vi "Teleop[Conflict 1].vi"(10 "Match Info":T1={"Autonomous Elapsed Seconds"=0.0, "TeleOp Elapsed Seconds"=0.0, "Disabled Elapsed Seconds"=0.0, "Visited Autonomous"=FALSE, "Visited TeleOp"=FALSE, "Visited Disabled"=FALSE, "Autonomous Settings"={"Autonomous Style"=enum."Independent", "VI Refnum"=refnum}}, 11 "Call Context":T2) -> ()   [LabVIEW 2016]
doc: "This VI is called for each TeleOp packet received from the DS where the robot is not disabled. It is often used to read from the joysticks and update I/O or to update setpoints for timed control loops. It should complete and return within 20 milliseconds or it may miss DS packets."
uses:
  <vilib>/Rock Robotics/WPI/DriverStation/WPI_DriverStationDerivedRobotMode.ctl
  <vilib>/Rock Robotics/WPI/DriverStation/WPI_DriverStationMatch Info.ctl
  <vilib>/Rock Robotics/Network Tables/NT Read Boolean.vi
  <vilib>/Rock Robotics/Network Tables/NT Read Number.vi
  <vilib>/Rock Robotics/WPI/Utilities/WPI_GetSetVariantRefNum.vi
  <vilib>/Rock Robotics/Network Tables/NT Write Boolean.vi
  <vilib>/Rock Robotics/Network Tables/NT Write Number.vi
  <vilib>/Rock Robotics/Network Tables/NT Write Boolean Array.vi
  <vilib>/Rock Robotics/Network Tables/NT Write Numeric Array.vi
  <vilib>/Rock Robotics/WPI/Solenoid/Deprecated/WPI_SolenoidSetBool.vi
  PDP Currents Variable.vi
panel:
  out "all currents (A) 2":dbl[](array[numeric])
  out "all currents (A)":dbl[](array[numeric])
  out "Enabled":bool
  out "Compressor Running":bool
  out "Sample Slider 0":dbl(slide) scale=0.0..5.0
  out "Sample Boolean 1":bool
  out "Sample Boolean 0":bool
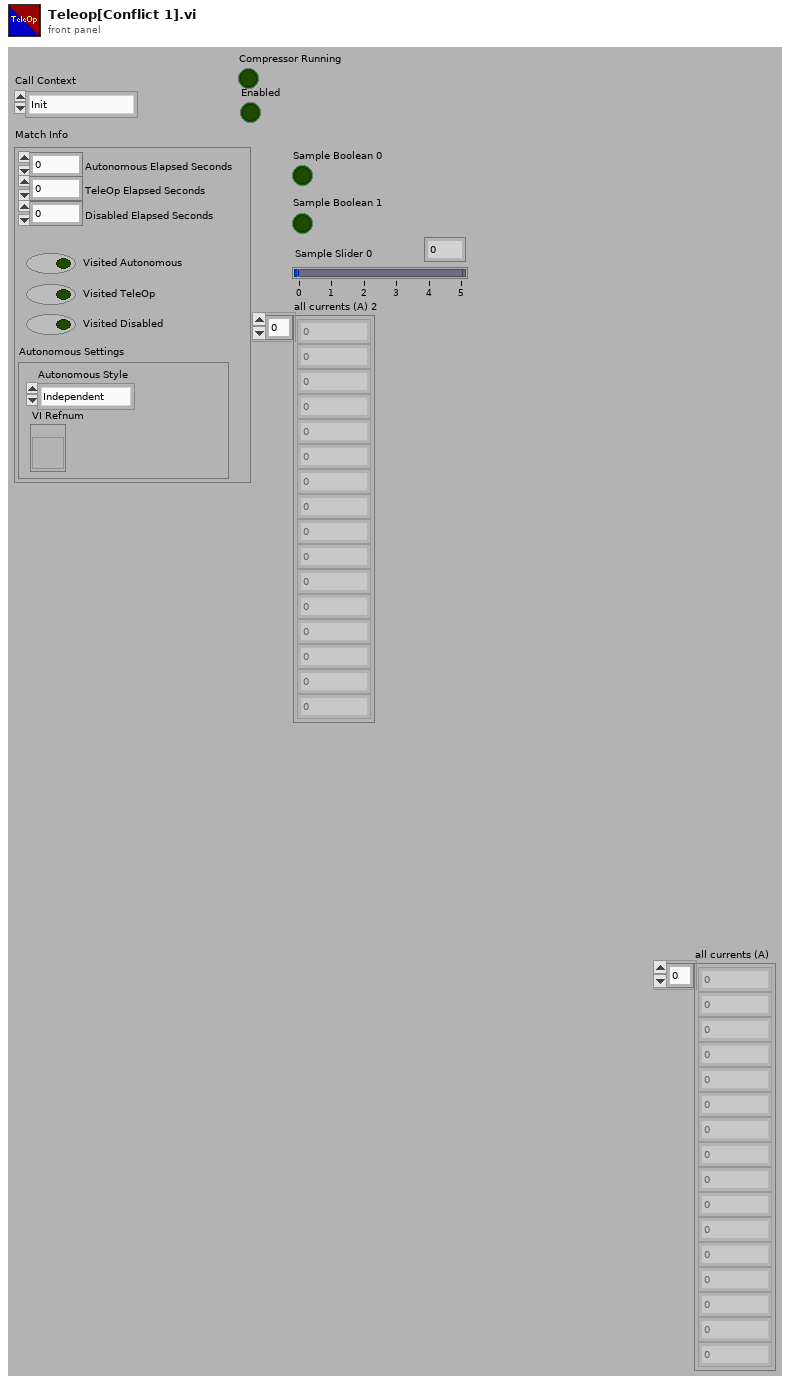
[diagram p1: front panel]
types:
  T1 = typedef "WPI_DriverStationMatch Info.ctl" = cluster{"Autonomous Elapsed Seconds":dbl, "TeleOp Elapsed Seconds":dbl, "Disabled Elapsed Seconds":dbl, "Visited Autonomous":bool, "Visited TeleOp":bool, "Visited Disabled":bool, "Autonomous Settings":cluster{"Autonomous Style":enum16{"Iterative", "Independent"}, "VI Refnum":refnum<vi>}}
  T2 = typedef "WPI_DriverStationDerivedRobotMode.ctl" = enum16{"Init", "Execute", "Stop"}
  T3 = typedef "WPI_JoystickDevRef.ctl" = cluster{"Device":T4}
  T4 = typedef "WPI_JoystickDeviceEnum.ctl" = enum16{"USB 0", "USB 1", "USB 2", "USB 3", "USB 4", "USB 5"}
  T5 = typedef "WPI_CompressorDevRef.ctl" = cluster{"DevStatus":errorcluster, "Pneumatics Control Module":u8}
  T6 = typedef "WPI_SolenoidDevRef.ctl" = cluster{"DevStatus":errorcluster, "Pneumatics Control Module":u8, "Forward Solenoid Channel":T7, "Reverse Solenoid Channel":T7}
  T7 = typedef "WPI_SolenoidChannel.ctl" = enum8{"Solenoid 0", "Solenoid 1", "Solenoid 2", "Solenoid 3", "Solenoid 4", "Solenoid 5", "Solenoid 6", "Solenoid 7", "Invalid"}
  T8 = typedef "WPI_SwitchDevRef.ctl" = cluster{"DevStatus":errorcluster, "DIO Channel":T9, "CntIndex":T10, "Normally Closed":bool}
  T9 = typedef "FPGA_DIOChannel.ctl" = enum8{"DIO 0", "DIO 1", "DIO 2", "DIO 3", "DIO 4", "DIO 5", "DIO 6", "DIO 7", "DIO 8", "DIO 9", "DIO MXP 0", "DIO MXP 1", "DIO MXP 2", "DIO MXP 3", "DIO MXP 4", "DIO MXP 5", "DIO MXP 6", "DIO MXP 7", "DIO MXP 8", "DIO MXP 9", "DIO MXP 10", "DIO MXP 11", "DIO MXP 12", "DIO MXP 13", "DIO MXP 14", "DIO MXP 15", "SPI Port CS1", "SPI Port CS2", "SPI Port CS3", "SPI Port MISO", "SPI Port MOSI", "Invalid"}
  T10 = typedef "FPGA_CounterCtrSystemIndex.ctl" = enum8{"Ctr 0", "Ctr 1", "Ctr 2", "Ctr 3", "Ctr 4", "Ctr 5", "Ctr 6", "Ctr 7", "Invalid"}
  T11 = typedef "WPI_MotorControlDeviceRef.ctl" = cluster{"DeviceStatus":errorcluster, "Type":T12, "PWM":cluster{"PWM Channel":T13, "DeadBand":T14}, "CAN":cluster{"Device Number":u8, "SetOutput VI Ref":variant, "GetOutput VI Ref":variant, "Enable VI Ref":variant, "Disable VI Ref":variant, "Data":variant}, "Invert":bool}
  T12 = typedef "WPI_MotorControlType.ctl" = enum16{"PWM", "CAN"}
  T13 = typedef "FPGA_DIOPWMChannel.ctl" = enum8{"PWM 0", "PWM 1", "PWM 2", "PWM 3", "PWM 4", "PWM 5", "PWM 6", "PWM 7", "PWM 8", "PWM 9", "PWM MXP 0", "PWM MXP 1", "PWM MXP 2", "PWM MXP 3", "PWM MXP 4", "PWM MXP 5", "PWM MXP 6", "PWM MXP 7", "PWM MXP 8", "PWM MXP 9", "Invalid"}
  T14 = typedef "WPI_PWMDeadband.ctl" = cluster{"Name":string, "maxPositivePwm":i32, "minPositivePwm":i32, "centerPwm":i32, "maxNegativePwm":i32, "minNegativePwm":i32, "angularRange":u16}
  T15 = typedef "WPI_RobotDriveDevRef.ctl" = cluster{"DevStatus":errorcluster, "Motors[]":T11[], "Square Inputs":bool, "Max Output":dbl}
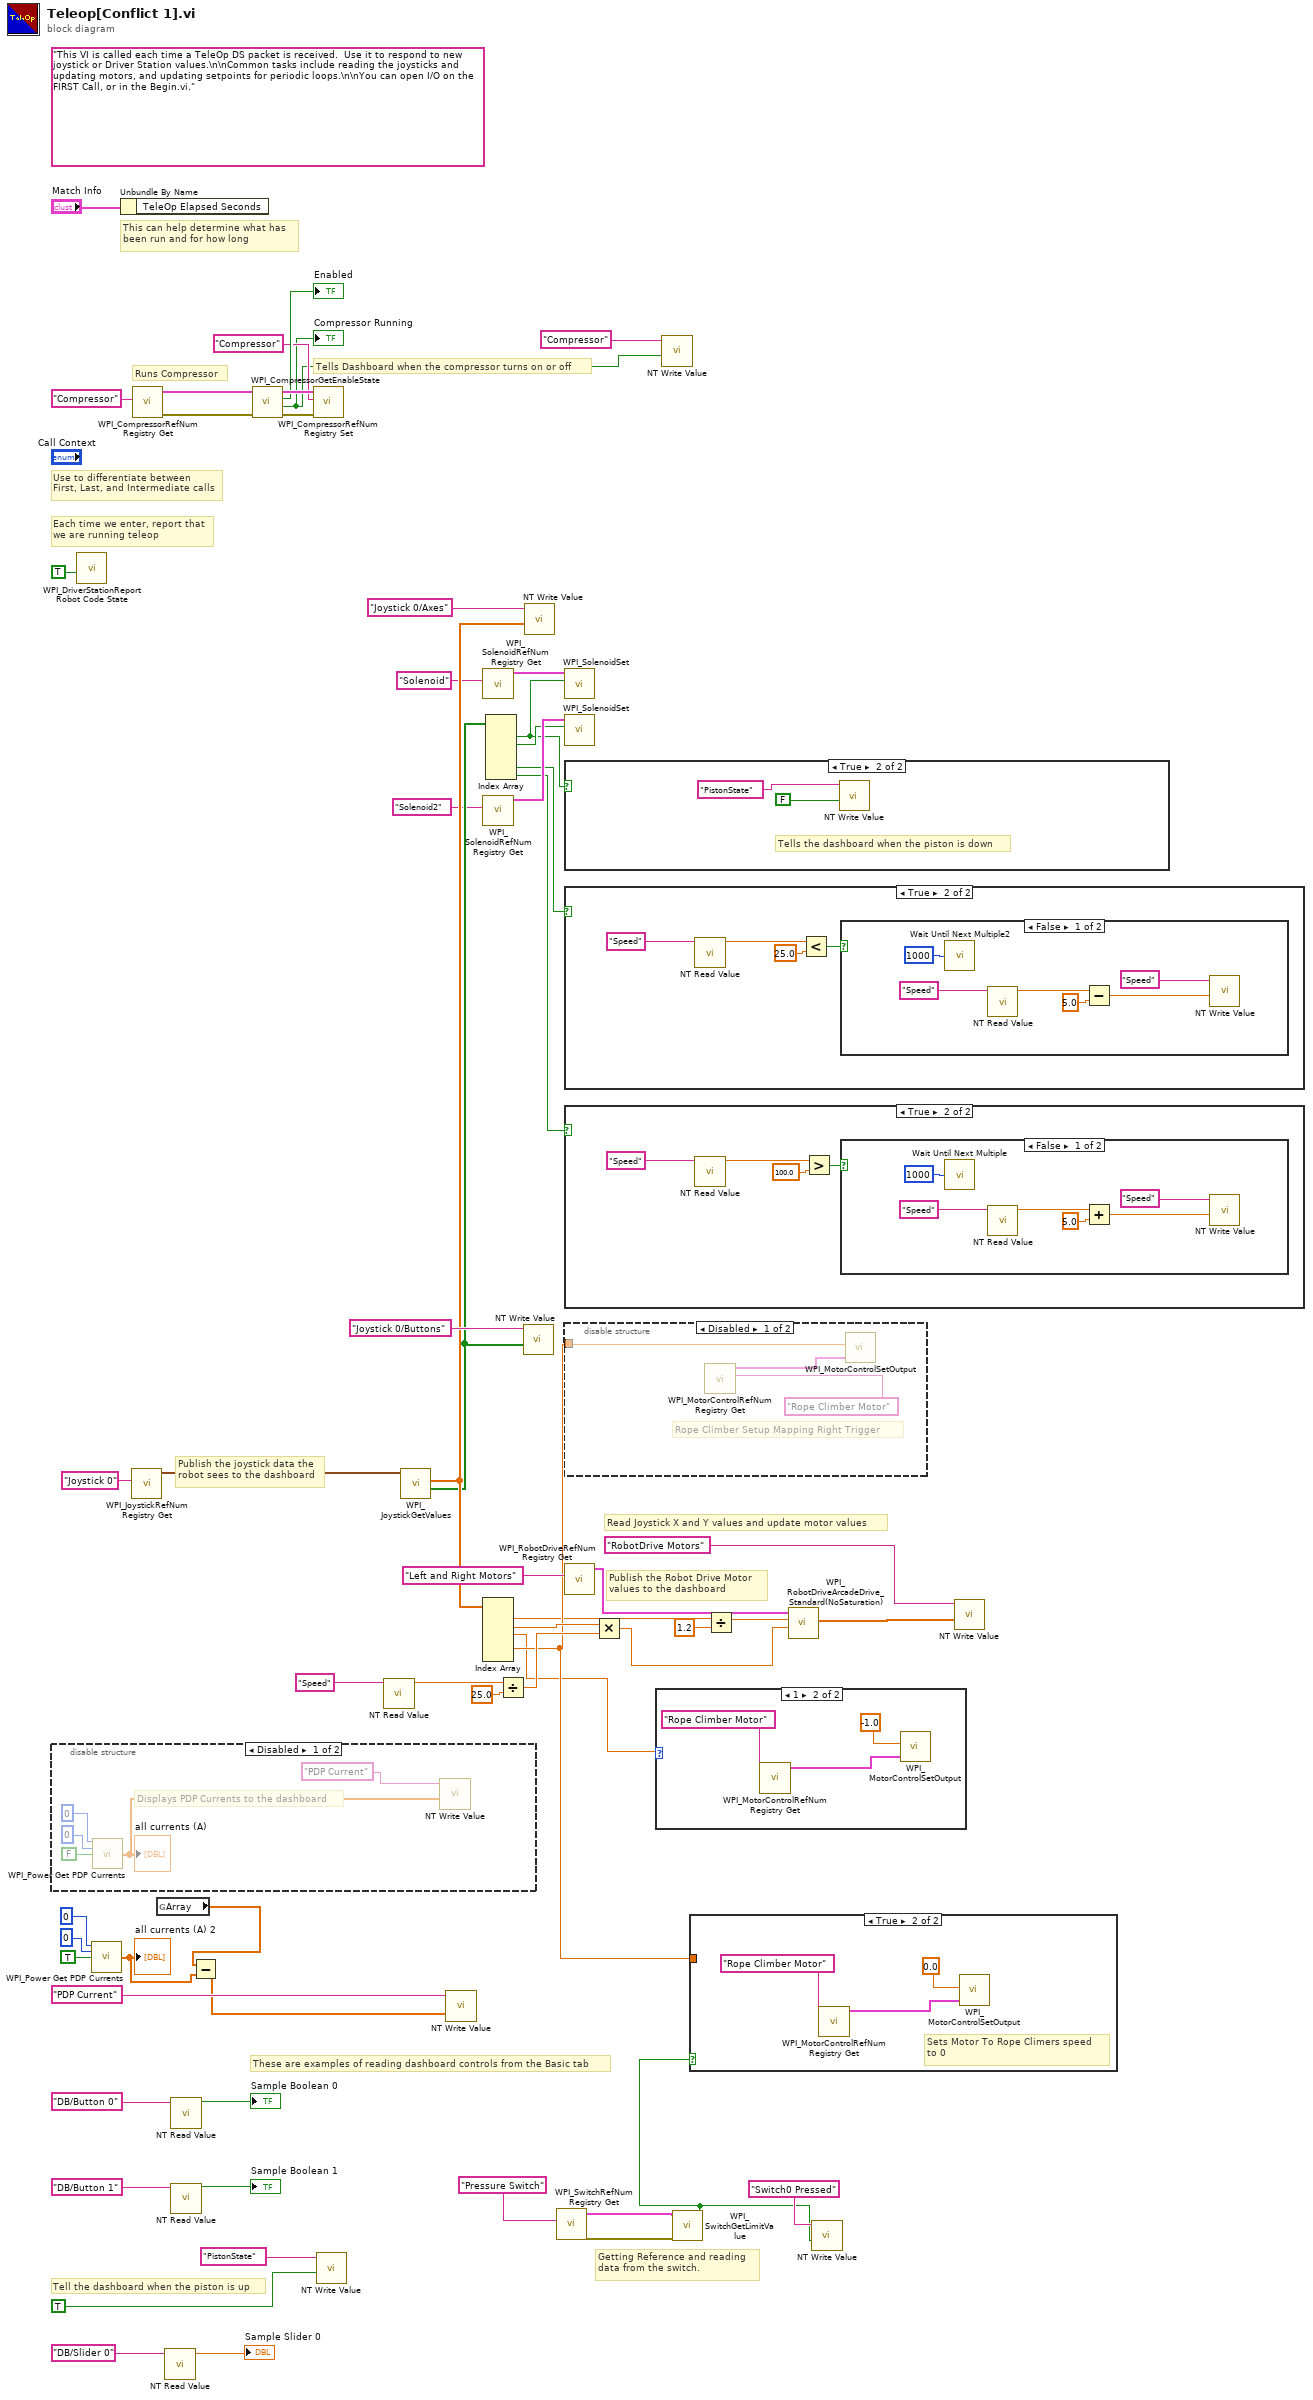
[diagram p0: block diagram]
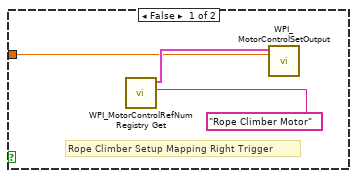
[diagram p4: hidden frame]
diagram:
  (unwired) "This VI is called each time a TeleOp DS packet is received.  Use it to respond to new joystick or Driver Station values.\n\nCommon tasks include reading the joysticks and updating motors, and updating setpoints for periodic loops.\n\nYou can open I/O on the FIRST Call, or in the Begin.vi."
  # "Getting Reference and reading \ndata from the switch."
  # "Tell the dashboard when the piston is up"
  # "Publish the joystick data the\nrobot sees to the dashboard"
  # "Publish the Robot Drive Motor\nvalues to the dashboard"
  # "Read Joystick X and Y values and update motor values"
  # "Tells Dashboard when the compressor turns on or off"
  # "Runs Compressor"
  # "These are examples of reading dashboard controls from the Basic tab"
  # "Each time we enter, report that\nwe are running teleop"
  # "Use to differentiate between\nFirst, Last, and Intermediate calls"
  # "This can help determine what has\nbeen run and for how long"
  n1 = disable-structure shown="Disabled" {
    frame Disabled {
      # "Displays PDP Currents to the dashboard"
      n2 = call <vilib>:"WPI_Power Get PDP Currents.vi"("Power Distribution Panel (0)"=u8 0, "PDP Channel"=0, "Tare Currents?"=FALSE) -> ("all currents (A)"=w63:dbl[])  [unwired: 10 in, 2 out]
      "all currents (A)" <- w63
      n3 = call-poly <vilib>:"NT Write Value.vi"("Numeric Array"=w63, "Name"="PDP Current") -> ()  [unwired: 9 in, 1 out]
    }
    frame Enabled {
    }
  }
  n4 = call <vilib>:"WPI_DriverStationReport Robot Code State.vi"("TeleOp"=TRUE ("Autonomous")) -> ()  [unwired: 10 in, 1 out]
  n5 = call <vilib>:"WPI_Power Get PDP Currents.vi"("Power Distribution Panel (0)"=u8 0, "PDP Channel"=0, "Tare Currents?"=TRUE) -> ("all currents (A)"=w13:dbl[])  [unwired: 10 in, 2 out]
  "all currents (A) 2" <- w13
  n6 = Unbundle By Name("Match Info") -> ()  [unwired: 1 out]
  n7 = call <vilib>:"WPI_JoystickRefNum Registry Get.vi"("refnum name"="Joystick 0") -> ("JoystickDevRef"=w40:T3)  [unwired: 1 in, 9 out]
  n8 = call <vilib>:"WPI_CompressorRefNum Registry Get.vi"("refnum name"="Compressor") -> ("error out"=w50:errorcluster, "CompressorDevRef"=w52:T5)  [unwired: 9 in]
  n9 = global read "PDP Currents Variable.vi" "Array"() -> (w11:dbl[])
  n10 = call-poly <vilib>:"NT Read Value.vi"("Name"="DB/Slider 0" ("refnum name")) -> ("Numeric"=→"Sample Slider 0":dbl)  [unwired: 9 in, 1 out]
  n11 = call-poly <vilib>:"NT Read Value.vi"("Name"="DB/Button 0" ("refnum name")) -> ("Boolean"=→"Sample Boolean 0":bool)  [unwired: 9 in, 1 out]
  n12 = call-poly <vilib>:"NT Read Value.vi"("Name"="DB/Button 1" ("refnum name")) -> ("Boolean"=→"Sample Boolean 1":bool)  [unwired: 9 in, 1 out]
  n13 = Subtract(x=w11, y=w13) -> (x-y=w12:dbl[])
  n14 = call <vilib>:"WPI_CompressorGetEnableState.vi"("error in (no error)"=w50, "CompressorDevRef"=w52) -> ("error out"=w49:errorcluster, "Compressor Running"=w44:bool, "Enabled"=→"Enabled":bool, "CompressorDevRef"=w51:T5)  [unwired: 6 in]
  "Compressor Running" <- w44
  n15 = call <vilib>:"WPI_CompressorRefNum Registry Set.vi"("error in (no error)"=w49, "refnum name"="Compressor", "CompressorDevRef"=w51) -> ()  [unwired: 7 in, 2 out]
  n16 = call-poly <vilib>:"NT Write Value.vi"("Boolean"=TRUE, "Name"="PistonState") -> ()  [unwired: 9 in, 1 out]
  n17 = call-poly <vilib>:"NT Read Value.vi"("Name"="Speed") -> ("Numeric"=w23:dbl)  [unwired: 9 in, 1 out]
  n18 = call <vilib>:"WPI_JoystickGetValues.vi"("JoystickDevRef"=w40) -> ("Buttons"=w34:bool[], "Axes"=w37:dbl[])  [unwired: 6 in, 3 out]
  n19 = call-poly <vilib>:"NT Write Value.vi"("Numeric Array"=w12, "Name"="PDP Current") -> ()  [unwired: 9 in, 1 out]
  n20 = call <vilib>:"WPI_SolenoidRefNum Registry Get.vi"("refnum name"="Solenoid") -> ("SolenoidDevRef"=w30:T6)  [unwired: 9 in, 1 out]
  n21 = call <vilib>:"WPI_SolenoidRefNum Registry Get.vi"("refnum name"="Solenoid2") -> ("SolenoidDevRef"=w32:T6)  [unwired: 9 in, 1 out]
  n22 = Index Array(array=w37) -> (element #2=w25:dbl, element #3=w4:dbl, element #4=w5:dbl, element #5=w1:dbl)  [unwired: 6 in, 2 out]
  n23 = Index Array(array=w34) -> (element #1=w28:bool, element #2=w29:bool, element #5=w18:bool, element #6=w19:bool)  [unwired: 6 in, 2 out]
  n24 = Divide(x=w23, y=25.0 ("x")) -> (x/y=w21:dbl)
  n25 = call-poly <vilib>:"NT Write Value.vi"("Boolean Array"=w34, "Name"="Joystick 0/Buttons") -> ()  [unwired: 9 in, 1 out]
  n26 = call-poly <vilib>:"NT Write Value.vi"("Numeric Array"=w37, "Name"="Joystick 0/Axes") -> ()  [unwired: 9 in, 1 out]
  n27 = call <vilib>:"WPI_SwitchRefNum Registry Get.vi"("refnum name"="Pressure Switch") -> ("error out"=w8:errorcluster, "SwitchDevRef"=w9:T8)  [unwired: 9 in]
  n28 = call-poly <vilib>:"WPI_SolenoidSet.vi"("Value"=w28, "SolenoidDevRef"=w30) -> ()  [unwired: 8 in, 2 out]
  n29 = call-poly <vilib>:"WPI_SolenoidSet.vi"("Value"=w29, "SolenoidDevRef"=w32) -> ()  [unwired: 8 in, 2 out]
  n30 = case shown="True" w28 {
    frame False {
    }
    frame True {
      # "Tells the dashboard when the piston is down"
      n31 = call-poly <vilib>:"NT Write Value.vi"("Boolean"=FALSE, "Name"="PistonState") -> ()  [unwired: 9 in, 1 out]
    }
  }
  n32 = case shown="True" w18 {
    frame False {
    }
    frame True {
      n33 = call-poly <vilib>:"NT Read Value.vi"("Name"="Speed") -> ("Numeric"=w70:dbl)  [unwired: 9 in, 1 out]
      n34 = Less?(x=w70, y=25.0) -> (x < y?=w68:bool)
      n35 = case shown="False" w68 {
        frame False {
          n36 = call "Wait Until Next Multiple2"("Count(mSec)"=u32 1000) -> ()  [unwired: 1 out]
          n37 = call-poly <vilib>:"NT Read Value.vi"("Name"="Speed") -> ("Numeric"=w76:dbl)  [unwired: 9 in, 1 out]
          n38 = Subtract(x=w76, y=5.0) -> (x-y=w74:dbl)
          n39 = call-poly <vilib>:"NT Write Value.vi"("Numeric"=w74, "Name"="Speed") -> ()  [unwired: 9 in, 1 out]
        }
        frame True {
        }
      }
    }
  }
  n40 = case shown="True" w19 {
    frame False {
    }
    frame True {
      n41 = call-poly <vilib>:"NT Read Value.vi"("Name"="Speed") -> ("Numeric"=w79:dbl)  [unwired: 9 in, 1 out]
      n42 = Greater?(x=w79, y=100.0) -> (0:w80:bool)
      n43 = case shown="False" w80 {
        frame False {
          n44 = call "Wait Until Next Multiple"("Count(mSec)"=u32 1000) -> ()  [unwired: 1 out]
          n45 = call-poly <vilib>:"NT Read Value.vi"("Name"="Speed") -> ("Numeric"=w83:dbl)  [unwired: 9 in, 1 out]
          n46 = Add(x=w83, y=5.0) -> (x+y=w85:dbl)
          n47 = call-poly <vilib>:"NT Write Value.vi"("Numeric"=w85, "Name"="Speed") -> ()  [unwired: 9 in, 1 out]
        }
        frame True {
        }
      }
    }
  }
  n48 = disable-structure shown="Disabled" {
    disable-tunnel: w5 -> [w88 _]
    frame Disabled {
      # "Rope Climber Setup Mapping Right Trigger"
      n49 = call <vilib>:"WPI_MotorControlRefNum Registry Get.vi"("refnum name"="Rope Climber Motor") -> ("MotorControlDevRef"=w89:T11)  [unwired: 9 in, 1 out]
      n50 = call <vilib>:"WPI_MotorControlSetOutput.vi"("Output"=w88, "MotorControlDevRef"=w89) -> ()  [unwired: 7 in, 3 out]
    }
    frame Enabled {
    }
  }
  n51 = call <vilib>:"WPI_RobotDriveRefNum Registry Get.vi"("refnum name"="Left and Right Motors") -> ("RobotDriveDevRef"=w42:T15)  [unwired: 1 in, 9 out]
  n52 = Multiply(x=w25, y=w21) -> (x*y=w20:dbl)
  n53 = case shown="1" w4 {
    frame 0, Default {
    }
    frame 1 {
      n54 = call <vilib>:"WPI_MotorControlRefNum Registry Get.vi"("refnum name"="Rope Climber Motor") -> ("MotorControlDevRef"=w93:T11)  [unwired: 9 in, 1 out]
      n55 = call <vilib>:"WPI_MotorControlSetOutput.vi"("Output"=-1.0 ("Motor Output"), "MotorControlDevRef"=w93) -> ()  [unwired: 7 in, 3 out]
    }
  }
  n56 = call-poly <vilib>:"NT Write Value.vi"("Boolean"=w44, "Name"="Compressor") -> ()  [unwired: 9 in, 1 out]
  n57 = call <vilib>:"WPI_SwitchGetLimitValue.vi"("error in (no error)"=w8, "SwitchDevRef"=w9) -> ("Switch Pressed"=w6:bool)  [unwired: 7 in, 2 out]
  n58 = case shown="True" w6 {
    tunnel: w5 -> [w94 _]
    frame False {
      # "Rope Climber Setup Mapping Right Trigger"
      n59 = call <vilib>:"WPI_MotorControlRefNum Registry Get.vi"("refnum name"="Rope Climber Motor") -> ("MotorControlDevRef"=w95:T11)  [unwired: 9 in, 1 out]
      n60 = call <vilib>:"WPI_MotorControlSetOutput.vi"("Output"=w94, "MotorControlDevRef"=w95) -> ()  [unwired: 7 in, 3 out]
    }
    frame True {
      # "Sets Motor To Rope Climers speed \nto 0"
      n61 = call <vilib>:"WPI_MotorControlRefNum Registry Get.vi"("refnum name"="Rope Climber Motor") -> ("MotorControlDevRef"=w99:T11)  [unwired: 9 in, 1 out]
      n62 = call <vilib>:"WPI_MotorControlSetOutput.vi"("Output"=0.0 ("Motor Output"), "MotorControlDevRef"=w99) -> ()  [unwired: 7 in, 3 out]
    }
  }
  n63 = Divide(x=w1, y=1.2) -> (x/y=w2:dbl)
  n64 = call <vilib>:"WPI_RobotDriveArcadeDrive_Standard(NoSaturation).vi"("Y axis value"=w20, "X axis value"=w2, "RobotDriveDevRef"=w42) -> ("Motor Values"=w36:dbl[])  [unwired: 1 in, 7 out]
  n65 = call-poly <vilib>:"NT Write Value.vi"("Boolean"=w6, "Name"="Switch0 Pressed") -> ()  [unwired: 9 in, 1 out]
  n66 = call-poly <vilib>:"NT Write Value.vi"("Numeric Array"=w36, "Name"="RobotDrive Motors") -> ()  [unwired: 9 in, 1 out]
